vi "Check If motor is rotating.vi"(8 "error in (no error)":errorcluster, 10 "No samples":u32, 11 "Encoder signal":digitalwaveform(waveform)) -> (0 "error out":errorcluster, 1 "Not rotating":bool, 2 "Zeros":bool)   [LabVIEW 2023]
uses:
  <vilib>/Waveform/DWDTOps.llb/DWDT Boolean Array to Digital.vi
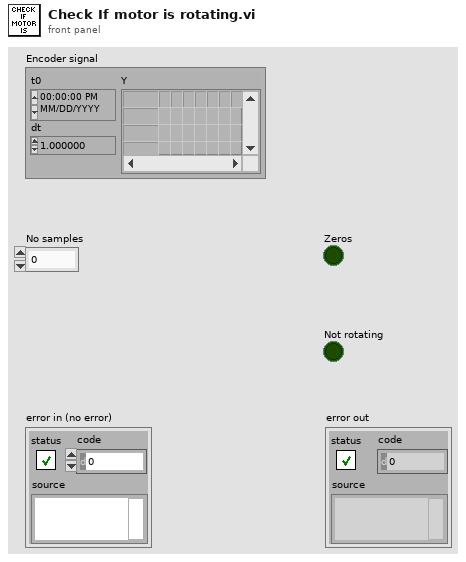
[diagram p1: front panel]
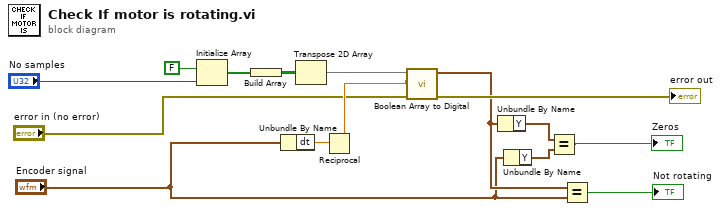
[diagram p0: block diagram]
diagram:
  n1 = Initialize Array(FALSE, "No samples") -> (w10:bool[])
  n2 = Build Array(w10) -> (w11:bool[][])
  n3 = Unbundle By Name("Encoder signal") -> ("dt"=w14:dbl)
  n4 = Transpose 2D Array(2D array=w11) -> (transposed array=w12:bool[][])
  n5 = Reciprocal(x=w14) -> (1/x=w15:dbl)
  n6 = call-poly <vilib>:"Boolean Array to Digital.vi"("error in (no error)"="error in (no error)", "sample rate"=w15, "boolean array"=w12) -> ("error out"=→"error out":errorcluster, "digital waveform"=w6:digitalwaveform)  [unwired: 7 in]
  n7 = Unbundle By Name(w6) -> ("Y"=w4:digitaldata)
  n8 = Unbundle By Name("Encoder signal") -> ("Y"=w3:digitaldata)
  n9 = Equal?(x=w4, y=w3) -> (x = y?=→"Zeros":bool)
  n10 = Equal?(x=w6, y="Encoder signal") -> (x = y?=→"Not rotating":bool)
